vi "Save Temp.vi"(8 "error in (no error)":errorcluster, 10 "temp file":string, 11 "Channel in":refnum<class "Channel.lvclass">) -> (0 "error out":errorcluster, 3 "Channel out":refnum<class "Channel.lvclass">)   [LabVIEW 2018, in "Channel.lvclass"]
uses:
  Channel.lvclass
  Channel.lvclass/Channel.ctl
  <vilib>/Utility/config.llb/Write Key (String).vi
  Interface/Interface.lvclass
  <vilib>/Utility/config.llb/NI_LVConfig.lvlib
panel:
  in  "Temp cluster":T1={"COOLER_POWER_STATUS"=0, "CURRENT_TEMPERATURE"=20} {"CURRENT_TEMPERATURE" min=0 max=0; "COOLER_POWER_STATUS" items=["Cooler OFF", "Cooler ON"]}
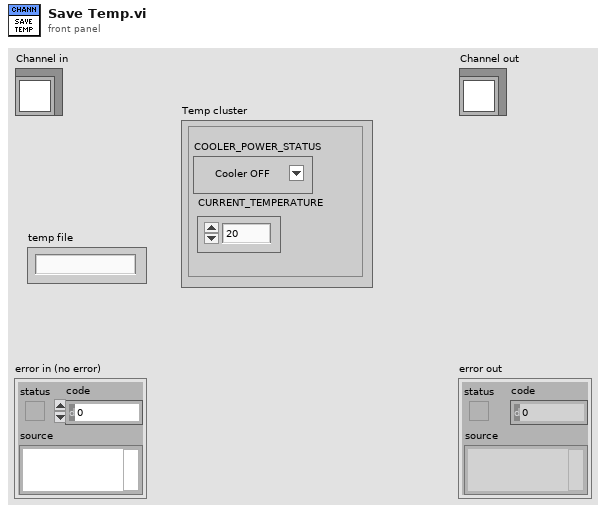
[diagram p1: front panel]
types:
  T1 = cluster{"COOLER_POWER_STATUS":i16, "CURRENT_TEMPERATURE":i8}
  T2 = typedef "NI_LVConfig.lvlib/Config Data RefNum.ctl" = refnum<k1>
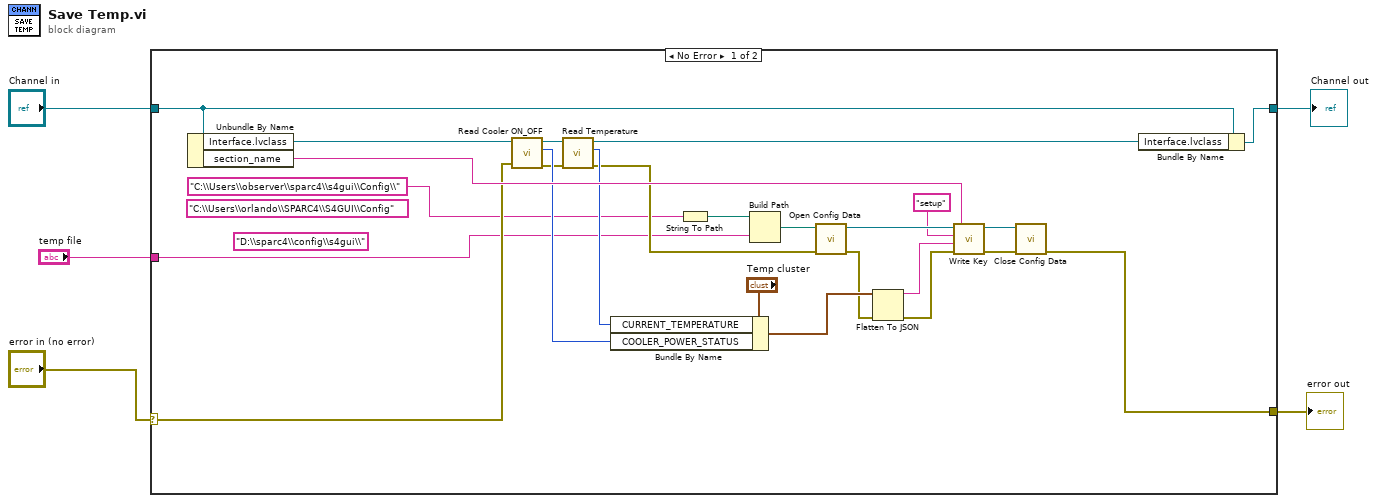
[diagram p0: block diagram]
diagram:
  n1 = case shown="No Error" "error in (no error)" {
    selector: "error in (no error)" -> [w12 w32]
    tunnel: [w21 w32] -> w1
    tunnel: [w25 w31] -> w2
    tunnel: "Channel in" -> [w26 w31]
    tunnel: "temp file" -> [w7 _]
    frame No Error {
      (unwired) "D:\\sparc4\\config\\s4gui\\" ("string")
      (unwired) "C:\\Users\\orlando\\SPARC4\\S4GUI\\Config"
      n2 = Unbundle By Name(w26) -> ("Interface.lvclass"=w24:refnum<class "Interface.lvclass">, "section_name"=w29:string)
      n3 = call-dynamic "Read Cooler ON_OFF.vi"("error in (no error)"=w12, "Interface in"=w24) -> ("error out"=w13:errorcluster, "Cooler ON/OFF"=w16:i16, "Interface out"=w20:refnum<class "Interface.lvclass">)  [unwired: 7 in]
      n4 = call-dynamic "Read Temperature.vi"("error in (no error)"=w13, "Interface in"=w20) -> ("error out"=w11:errorcluster, "Temperature"=w15:i8, "Interface out"=w19:refnum<class "Interface.lvclass">)  [unwired: 7 in]
      n5 = Bundle By Name(cluster="Temp cluster", "CURRENT_TEMPERATURE"=w15, "COOLER_POWER_STATUS"=w16) -> (w14:T1)
      n6 = String To Path(string="C:\\Users\\observer\\sparc4\\s4gui\\Config\\") -> (path=w8:path)
      n7 = Build Path(base path=w8, name or relative path=w7) -> (appended path=w30:path)
      n8 = call <vilib>:"Open Config Data.vi"("error in (no error)"=w11, "configuration file path"=w30) -> ("error out"=w10:errorcluster, "refnum"=w28:T2)  [unwired: 7 in, 1 out]
      n9 = Flatten To JSON(anything=w14, error in (no error)=w10) -> (JSON string=w17:string, 11:w9:errorcluster)  [unwired: 1 in]
      n10 = call-poly <vilib>:"Write Key.vi"("section"=w29, "error in (no error)"=w9, "value"=w17, "key"="setup", "refnum"=w28) -> ("error out"=w22:errorcluster, "refnum out"=w23:T2)  [unwired: 4 in, 1 out]
      n11 = call <vilib>:"Close Config Data.vi"("error in (no error)"=w22, "refnum"=w23) -> ("error out"=w21:errorcluster)  [unwired: 8 in, 1 out]
      n12 = Bundle By Name(cluster=w26, "Interface.lvclass"=w19) -> (w25:refnum<class "Channel.lvclass">)
    }
    frame Error {
    }
  }
  "error out" <- w1
  "Channel out" <- w2
